vi "Evaluate Targets for Shooting.vi"(7 "Distance Method":u16(ring)=2 items=["Default", "Center Calculations", "Hybrid"], 8 "Camera Distance\nfrom Ground (in)":dbl, 9 "Maximum Shooting Distance":dbl, 10 "More Detection":T1(array[cluster])) -> (3 "What to do":string)   [LabVIEW 2015]
panel:
  out "Not Center":bool
  out "Too Far":bool
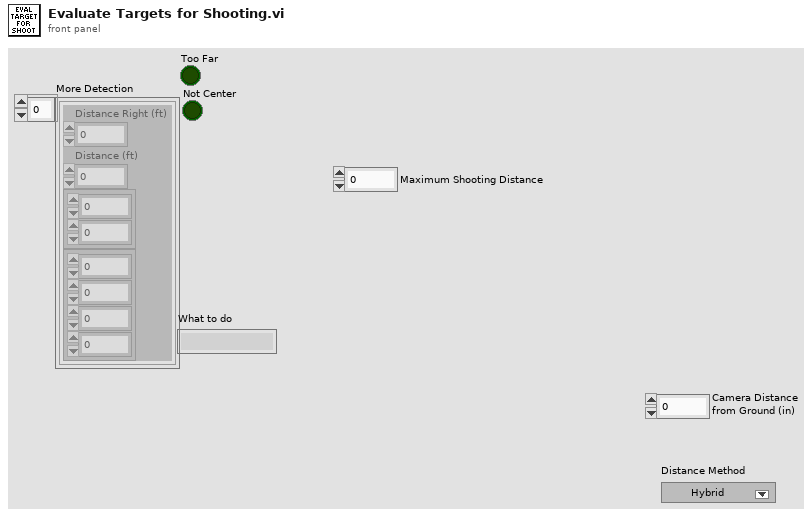
[diagram p1: front panel]
types:
  T1 = cluster{"Distance Right (ft)":dbl, "Distance (ft)":dbl, cluster{dbl, dbl}, cluster{dbl, dbl, dbl, dbl}}[]
  T2 = cluster{"Distance Right (ft)":dbl, "Distance (ft)":dbl, cluster{dbl, dbl}, cluster{dbl, dbl, dbl, dbl}}
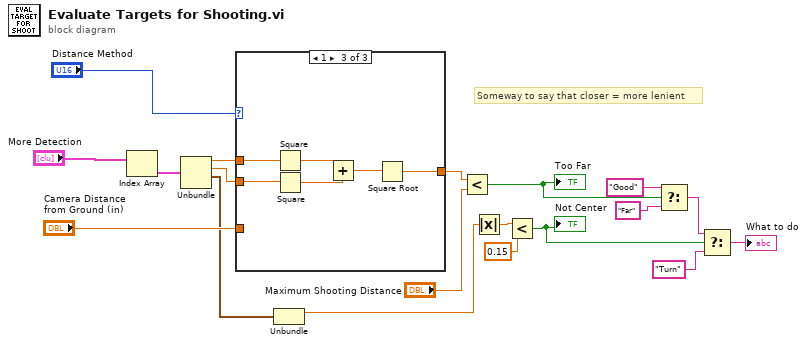
[diagram p0: block diagram]
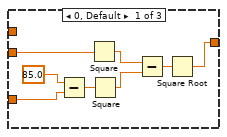
[diagram p2: hidden frame]
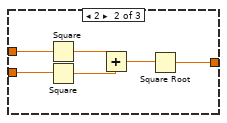
[diagram p3: hidden frame]
diagram:
  # "Someway to say that closer = more lenient"
  n1 = Index Array(array="More Detection") -> (element=w17:T2)  [unwired: 1 in]
  n2 = Unbundle(w17) -> ("Distance Right (ft)"=w16:dbl, "Distance (ft)"=w15:dbl, w11:cluster{dbl, dbl})  [unwired: 1 out]
  n3 = case shown="1" "Distance Method" {
    tunnel: w16 -> [_ w30 w36]
    tunnel: w15 -> [w27 w29 w35]
    tunnel: "Camera Distance\nfrom Ground (in)" -> [w24 _ _]
    tunnel: [w20 w28 w34] -> w13
    frame 0, Default {
      n4 = Subtract(x=85.0, y=w24) -> (x-y=w23:dbl)
      n5 = Square(x=w27) -> (x^2=w26:dbl)
      n6 = Square(x=w23) -> (x^2=w22:dbl)
      n7 = Subtract(x=w26, y=w22) -> (x-y=w21:dbl)
      n8 = Square Root(x=w21) -> (sqrt(x)=w20:dbl)
    }
    frame 2 {
      n9 = Square(x=w30) -> (x^2=w33:dbl)
      n10 = Square(x=w29) -> (x^2=w32:dbl)
      n11 = Add(x=w33, y=w32) -> (x+y=w31:dbl)
      n12 = Square Root(x=w31) -> (sqrt(x)=w28:dbl)
    }
    frame 1 {
      n13 = Square(x=w36) -> (x^2=w39:dbl)
      n14 = Square(x=w35) -> (x^2=w38:dbl)
      n15 = Add(x=w39, y=w38) -> (x+y=w37:dbl)
      n16 = Square Root(x=w37) -> (sqrt(x)=w34:dbl)
    }
  }
  n17 = Unbundle(w11) -> (w10:dbl)  [unwired: 1 out]
  n18 = Less?(x=w13, y="Maximum Shooting Distance") -> (x < y?=w7:bool)
  "Too Far" <- w7
  n19 = Absolute Value(x=w10) -> (abs(x)=w9:dbl)
  n20 = Less?(x=w9, y=0.15) -> (x < y?=w4:bool)
  "Not Center" <- w4
  n21 = Select(t="Good", s=w7, f="Far") -> (s? t:f=w2:string)
  n22 = Select(t=w2, s=w4, f="Turn") -> (s? t:f=→"What to do":string)
